vi "Create New RESTful Web Service from Build Object.vi"(8 "error in (no error)":errorcluster, 9 "Build Path":path, 10 "buildSpecName":string, 11 "buildObject":T1) -> (0 "error out":errorcluster, 3 "RESTful out":refnum<class "NI_AB_API_RESTful.lvclass">)   [LabVIEW 2020, in "NI_AB_API_RESTful.lvclass"]
uses:
  <vilib>/AppBuilder/AB_API/RESTful/NI_AB_API_RESTful.lvclass
  <vilib>/AppBuilder/AB_API/RESTful/NI_AB_API_RESTful.lvclass/NI_AB_API_RESTful.ctl
  <vilib>/AppBuilder/AB_API/Build/NI_AB_API_Build.lvclass
  <vilib>/AppBuilder/AB_Classes/RESTful/AB_RESTfulWebService.lvclass
  e:/builds/penguin/labview/branches/2020/dev/dist/vi.lib/AppBuilder/AB_Classes/WebService/AB_WebService.lvclass
  e:/builds/penguin/labview/branches/2020/dev/dist/vi.lib/AppBuilder/AB_Classes/TargetFile/AB_Targetfile.lvclass
  e:/builds/penguin/labview/branches/2020/dev/dist/vi.lib/AppBuilder/AB_Classes/Build/AB_Build.lvclass
  e:/builds/penguin/labview/branches/2020/dev/dist/vi.lib/AppBuilder/AB_Classes/RESTful/AB_RESTfulWebService.lvclass
  e:/builds/penguin/labview/branches/2020/dev/dist/vi.lib/AppBuilder/AB_API/Targetfile/NI_AB_API_Targetfile.lvclass
  e:/builds/penguin/labview/branches/2020/dev/dist/vi.lib/AppBuilder/AB_API/Build/NI_AB_API_Build.lvclass
  e:/builds/penguin/labview/branches/2020/dev/dist/vi.lib/AppBuilder/AB_API/RESTful/NI_AB_API_RESTful.lvclass
  <resource>/Framework/Providers/API/ItemRef.ctl
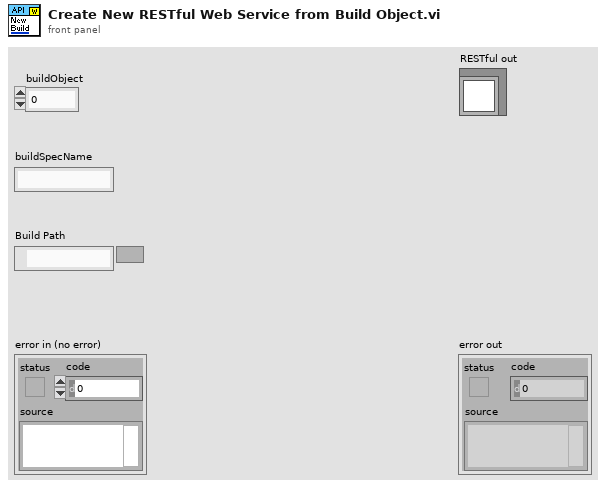
[diagram p1: front panel]
types:
  T1 = typedef "ItemRef.ctl" = u64
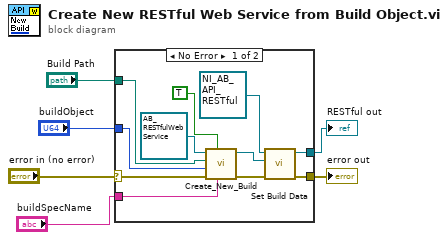
[diagram p0: block diagram]
diagram:
  n1 = case shown="No Error" "error in (no error)" {
    selector: "error in (no error)" -> [w11 w18]
    tunnel: [w8 w18] -> w5
    tunnel: [w9 _] -> w4
    tunnel: "buildObject" -> [w12 _]
    tunnel: "Build Path" -> [w10 _]
    tunnel: "buildSpecName" -> [w7 _]
    frame No Error {
      n2 = call-dynamic "Create_New_Build.vi"("buildSpecName"=w7, "Programmatic? (false)"=TRUE, "error in (no error)"=w11, "buildObject"=w12, "Destination Path"=w10, "AB_WebService in"=refnum<class "AB_RESTfulWebService.lvclass"> refnum ("AB_RESTfulWebService.lvclass")) -> ("error out"=w16:errorcluster, "AB_WebService out"=w15:refnum<class "AB_RESTfulWebService.lvclass">)  [unwired: 4 in]
      n3 = call <vilib>:"Set Build Data.vi"("error in (no error)"=w16, "AB_Build.lvclass"=w15, "NI_AB_API_Build in"=refnum<class "NI_AB_API_RESTful.lvclass"> refnum ("AB_API_SDIST.lvclass")) -> ("error out"=w8:errorcluster, "NI_AB_API_Build out"=w9:refnum<class "NI_AB_API_RESTful.lvclass">)  [unwired: 7 in]
    }
    frame Error {
    }
  }
  "error out" <- w5
  "RESTful out" <- w4
